vi "SendMeasureCommand (SubVI).vi"(8 "error in (no error)":errorcluster) -> (0 "error out":errorcluster, 2 "Command Sent?":bool)   [LabVIEW 2019]
doc: "Sends a command to the Machine instructing it to start its measurement routine.\nReturns a boolean TRUE or FALSE depending on whether the command was sent succesfully.\n\nFor more information:\nhttps://www.youtube.com/watch?v=oHg5SJYRHA0"
panel:
  # "Sends a command to the Machine \ninstructing it to start its measurement\nroutine. Returns a boolean TRUE or \nFALSE depending on whether the \ncommand was sent succesfully.\n\nFor more information:\nhttps://www.youtube.com/watch?v=oHg5SJYRHA0"
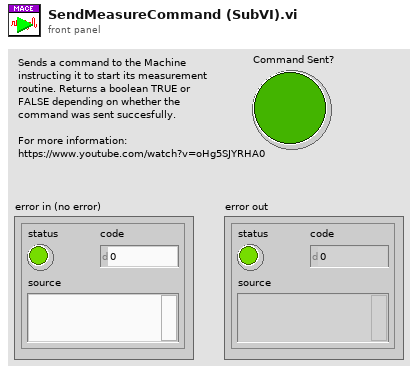
[diagram p1: front panel]
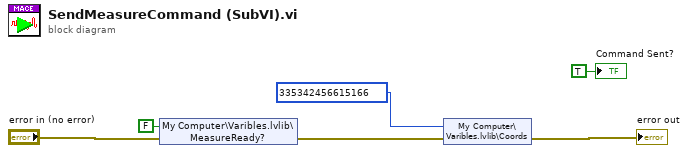
[diagram p0: block diagram]
diagram:
  n1 = shared-variable "My Computer\\Varibles.lvlib\\MeasureReady?"(FALSE ("MeasureReady?"), error in="error in (no error)") -> (error out=w1:errorcluster)
  n2 = shared-variable "My Computer\\Varibles.lvlib\\Coords"(u64 335342456615166 ("Coords"), error in=w1) -> (error out=→"error out":errorcluster)
  "Command Sent?" <- TRUE ("Command Sent?")
